vi "Get Variant.vi"(8 "error in (no error)":errorcluster, 11 "int32 in":refnum<class "sint64.lvclass">) -> (0 "error out":errorcluster, 2 "Variant":variant, 3 "int32 out":refnum<class "sint64.lvclass">)   [LabVIEW 2020, in "Protobuf RAW.lvlib" / "sint64.lvclass"]
uses:
  sint64.lvclass
  sint64.lvclass/sint64.ctl
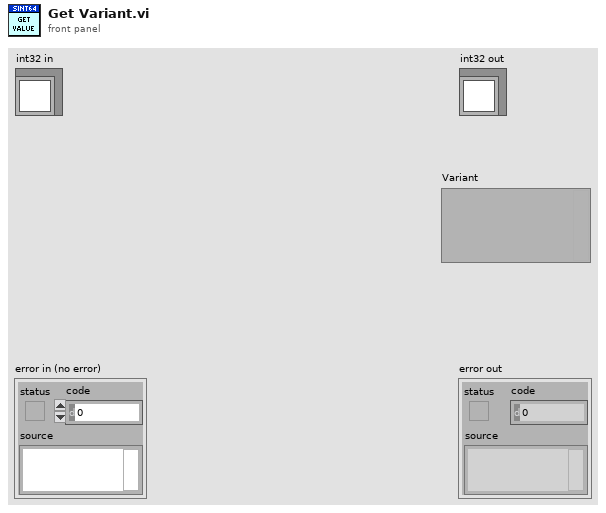
[diagram p1: front panel]
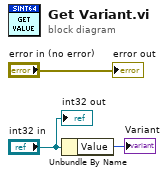
[diagram p0: block diagram]
diagram:
  n1 = Unbundle By Name("int32 in") -> ("Value"=→"Variant":i64)
  "error out" <- "error in (no error)"
  "int32 out" <- "int32 in"
